vi "Fahrenheit.vi"(4 "Celsius temperature":dbl) -> (1 "Fahrenheit temperature":dbl)   [LabVIEW 2014]
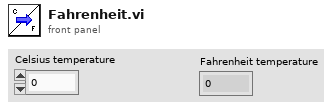
[diagram p1: front panel]
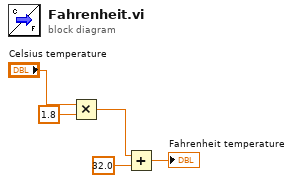
[diagram p0: block diagram]
diagram:
  n1 = Multiply(x="Celsius temperature", y=1.8) -> (x*y=w3:dbl)
  n2 = Add(x=w3, y=32.0) -> (x+y=→"Fahrenheit temperature":dbl)
